vi "ConfigDa.vi"(0 "Pump_1AI_1DO_2DI in":refnum<class "Engine_1DO_2DI.lvclass">, 11 "error in (no error)":errorcluster) -> (4 "Pump_1AI_1DO_2DI out":refnum<class "Engine_1DO_2DI.lvclass">, 15 "error out":errorcluster)   [LabVIEW 2019, in "Engine_1DO_2DI.lvclass"]
uses:
  Engine_1DO_2DI.lvclass
  D:/GIT H4000/H4000/src/Proccess_class/Proccess.lvclass
  Proccess_class/TAGs.ctl
  TypeDef/bool_setting.ctl
  DA_class/DA.lvclass
  Proccess_class/Proccess.lvclass/Proccess.ctl
  Engine_1DO_2DI.lvclass/Engine_1DO_2DI.ctl
  Proccess_class/Proccess.lvclass
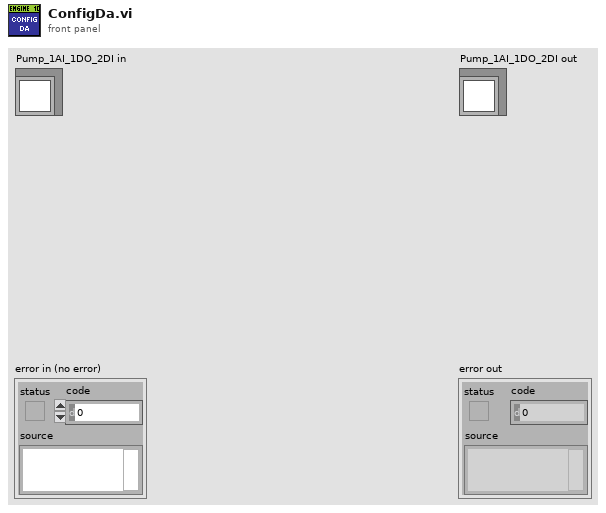
[diagram p1: front panel]
types:
  T1 = typedef "bool_setting.ctl" = cluster{"TON_ms":u32, "TOFF_ms":u32}
  T2 = typedef "Proccess.lvclass/TAGs.ctl" = cluster{"TAG":string, "PTAG":string, "DESC":string}
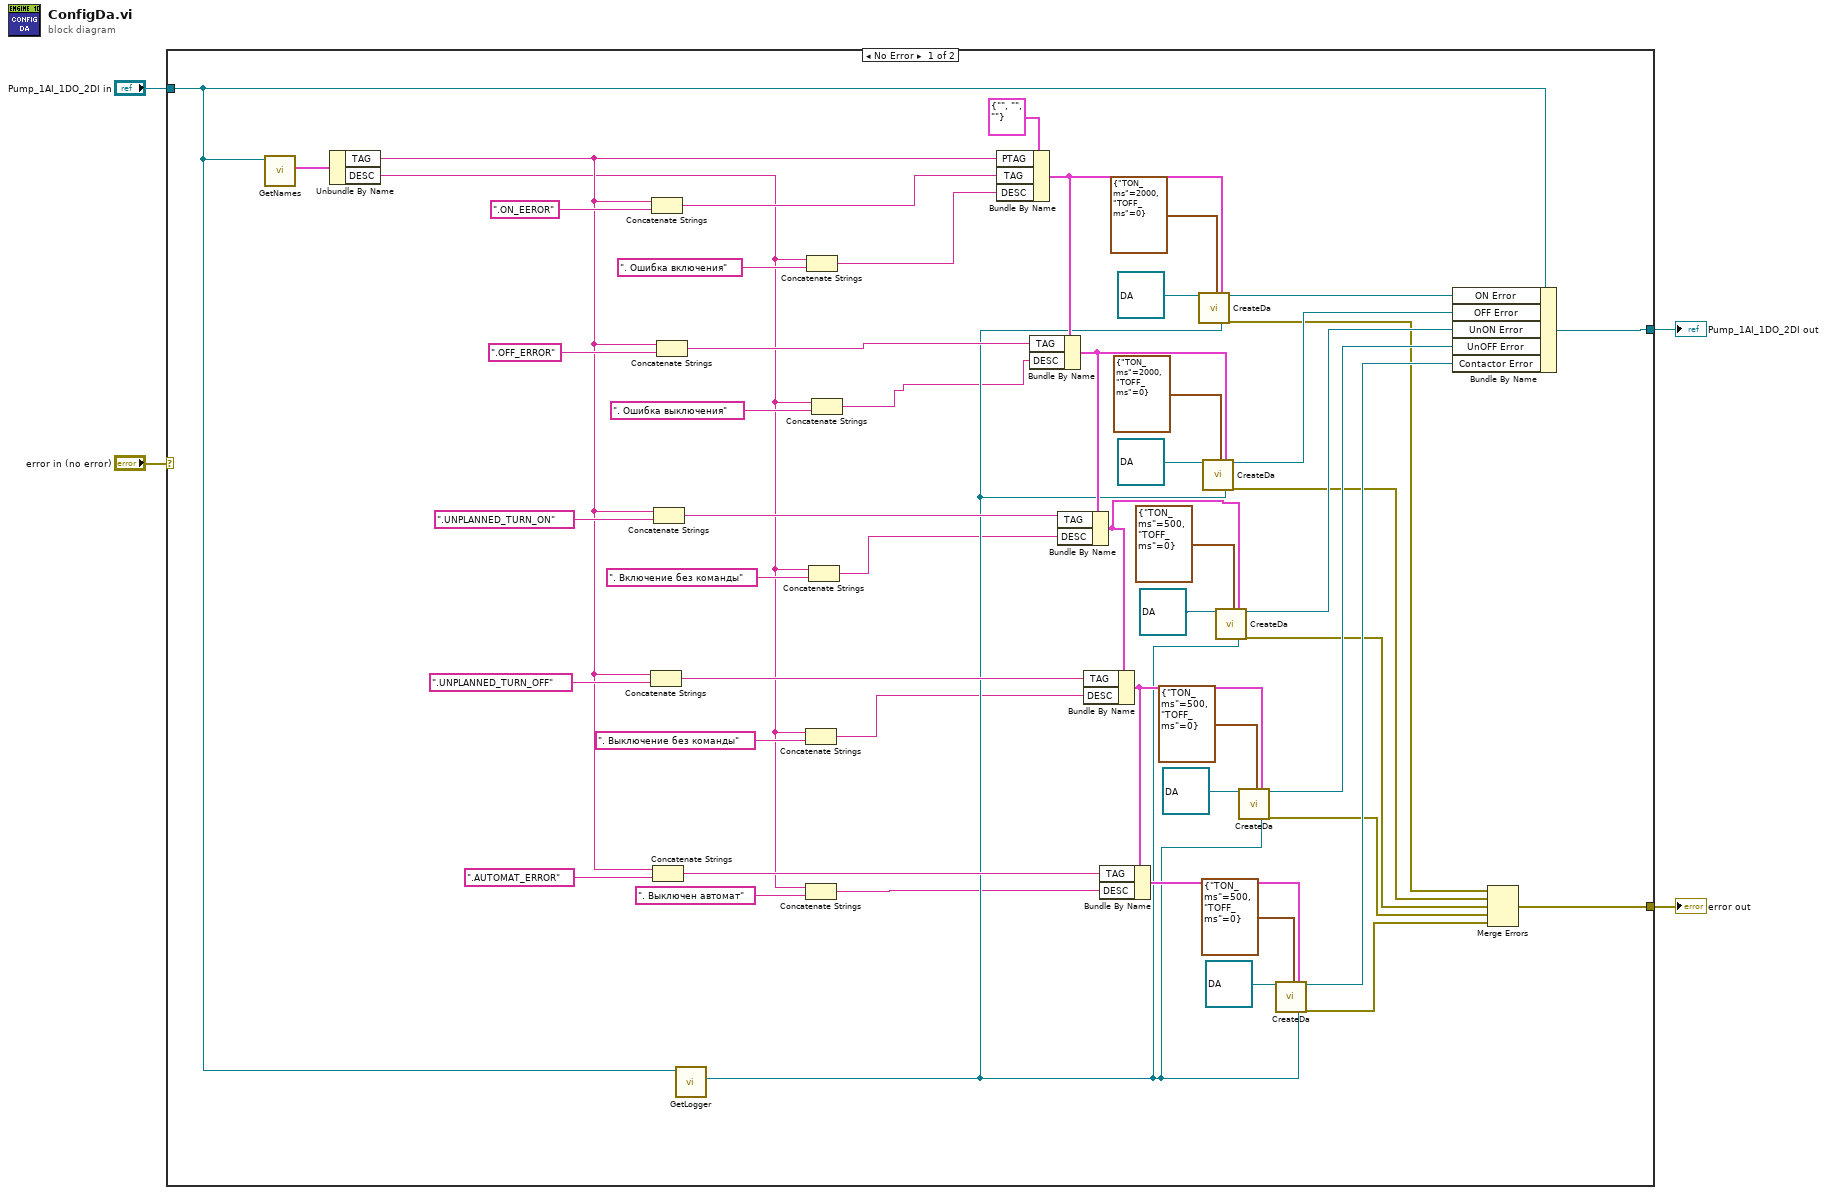
[diagram p0: block diagram]
diagram:
  n1 = case shown="No Error" "error in (no error)" {
    selector: "error in (no error)" -> [_ w59]
    tunnel: [w16 w59] -> w3
    tunnel: [w57 w58] -> w1
    tunnel: "Pump_1AI_1DO_2DI in" -> [w56 w58]
    frame No Error {
      n2 = call "GetNames.vi"("Proccess in"=w56) -> ("Tags"=w51:T2)  [unwired: 10 in]
      n3 = Unbundle By Name(w51) -> ("TAG"=w45:string, "DESC"=w10:string)
      n4 = Concatenate Strings(w45, ".UNPLANNED_TURN_OFF" ("string")) -> (w31:string)
      n5 = Concatenate Strings(w45, ".ON_EEROR" ("string")) -> (w48:string)
      n6 = Concatenate Strings(w45, ".AUTOMAT_ERROR" ("string")) -> (w24:string)
      n7 = Concatenate Strings(w45, ".UNPLANNED_TURN_ON" ("string")) -> (w36:string)
      n8 = Concatenate Strings(w45, ".OFF_ERROR" ("string")) -> (w40:string)
      n9 = call "GetLogger.vi"("Proccess in"=w56) -> ("Logger"=w22:refnum<class "Logger.lvclass">)  [unwired: 10 in]
      n10 = Concatenate Strings(w10, ". Выключение без команды" ("string")) -> (w6:string)
      n11 = Concatenate Strings(w10, ". Выключен автомат" ("string")) -> (w5:string)
      n12 = Concatenate Strings(w10, ". Ошибка включения" ("string")) -> (w9:string)
      n13 = Concatenate Strings(w10, ". Включение без команды" ("string")) -> (w7:string)
      n14 = Concatenate Strings(w10, ". Ошибка выключения" ("string")) -> (w8:string)
      n15 = Bundle By Name(cluster=T2 {"TAG"="", "PTAG"="", "DESC"=""} ("Tags"), "PTAG"=w45, "TAG"=w48, "DESC"=w9) -> (w41:T2)
      n16 = Bundle By Name(cluster=w41, "TAG"=w40, "DESC"=w8) -> (w35:T2)
      n17 = Bundle By Name(cluster=w35, "TAG"=w36, "DESC"=w7) -> (w30:T2)
      n18 = Bundle By Name(cluster=w30, "TAG"=w31, "DESC"=w6) -> (w25:T2)
      n19 = Bundle By Name(cluster=w25, "TAG"=w24, "DESC"=w5) -> (w28:T2)
      n20 = call "CreateDa.vi"("Sig_DA in"=refnum<class "DA.lvclass"> refnum ("Sig_DA"), "bool_setting"=T1 {"TON_ms"=2000, "TOFF_ms"=0}, "Tags"=w41, "Logger"=w22) -> ("Sig_DA out"=w43:refnum<class "DA.lvclass">, "error out"=w17:errorcluster)  [unwired: 14 in]
      n21 = call "CreateDa.vi"("Sig_DA in"=refnum<class "DA.lvclass"> refnum ("Sig_DA"), "bool_setting"=T1 {"TON_ms"=2000, "TOFF_ms"=0}, "Tags"=w35, "Logger"=w22) -> ("Sig_DA out"=w42:refnum<class "DA.lvclass">, "error out"=w18:errorcluster)  [unwired: 14 in]
      n22 = call "CreateDa.vi"("Sig_DA in"=refnum<class "DA.lvclass"> refnum ("Sig_DA"), "bool_setting"=T1 {"TON_ms"=500, "TOFF_ms"=0}, "Tags"=w30, "Logger"=w22) -> ("Sig_DA out"=w34:refnum<class "DA.lvclass">, "error out"=w19:errorcluster)  [unwired: 14 in]
      n23 = call "CreateDa.vi"("Sig_DA in"=refnum<class "DA.lvclass"> refnum ("Sig_DA"), "bool_setting"=T1 {"TON_ms"=500, "TOFF_ms"=0}, "Tags"=w25, "Logger"=w22) -> ("Sig_DA out"=w29:refnum<class "DA.lvclass">, "error out"=w20:errorcluster)  [unwired: 14 in]
      n24 = call "CreateDa.vi"("Sig_DA in"=refnum<class "DA.lvclass"> refnum ("Sig_DA"), "bool_setting"=T1 {"TON_ms"=500, "TOFF_ms"=0}, "Tags"=w28, "Logger"=w22) -> ("Sig_DA out"=w23:refnum<class "DA.lvclass">, "error out"=w21:errorcluster)  [unwired: 14 in]
      n25 = Bundle By Name(cluster=w56, "ON Error"=w43, "OFF Error"=w42, "UnON Error"=w34, "UnOFF Error"=w29, "Contactor Error"=w23) -> (w57:refnum<class "Engine_1DO_2DI.lvclass">)
      n26 = Merge Errors(w17, w18, w19, w20, w21) -> (w16:errorcluster)
    }
    frame Error {
    }
  }
  "error out" <- w3
  "Pump_1AI_1DO_2DI out" <- w1
